vi "direction safety.vi"(2 "Min Rate":dbl, 3 "Desired Rate":dbl, 4 "Encoder Rate":dbl) -> (0 "Encoder Directional Issue":bool, 1 "Super Safe Rate":dbl)   [LabVIEW 2013]
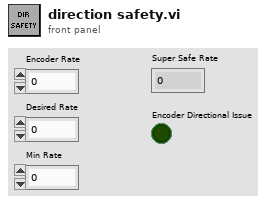
[diagram p1: front panel]
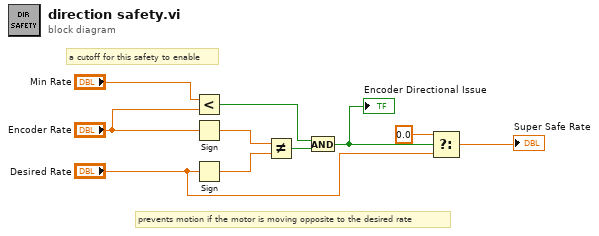
[diagram p0: block diagram]
diagram:
  # "prevents motion if the motor is moving opposite to the desired rate"
  # "a cutoff for this safety to enable"
  n1 = Less?(x="Min Rate", y="Encoder Rate") -> (x < y?=w2:bool)
  n2 = Sign(1:"Encoder Rate") -> (0:w8:dbl)
  n3 = Sign(1:"Desired Rate") -> (0:w7:dbl)
  n4 = Not Equal?(x=w8, y=w7) -> (x != y?=w3:bool)
  n5 = And(x=w2, y=w3) -> (x .and. y?=w1:bool)
  "Encoder Directional Issue" <- w1
  n6 = Select(t=0.0, s=w1, f="Desired Rate") -> (s? t:f=→"Super Safe Rate":dbl)
